vi "read_params.vi"(8 "error in (no error)":errorcluster, 11 "OPTICS in":refnum<class "OPTICS.lvclass">) -> (0 "error out":errorcluster, 2 "params":T1={"min_samples"=5.0, "max_eps"=inf, "metric"="euclidean", "p"=2.0, "cluster_method"="xi", "eps"={"eps_type"="None", "eps_float"=0.0}, "xi"=0.05, "predecessor_correction"=TRUE, "min_cluster_size"={"min_cluster_size_type"="None", "min_cluster_size_int"=1.0, "min_cluster_size_float"=0.0}, "algorithm"="auto", "leaf_size"=30.0, "n_jobs"=1.0}, 3 "OPTICS out":refnum<class "OPTICS.lvclass">)   [LabVIEW 2020, in "OPTICS.lvclass"]
uses:
  OPTICS.lvclass
  Controls/optics_params.ctl
  OPTICS.lvclass/OPTICS.ctl
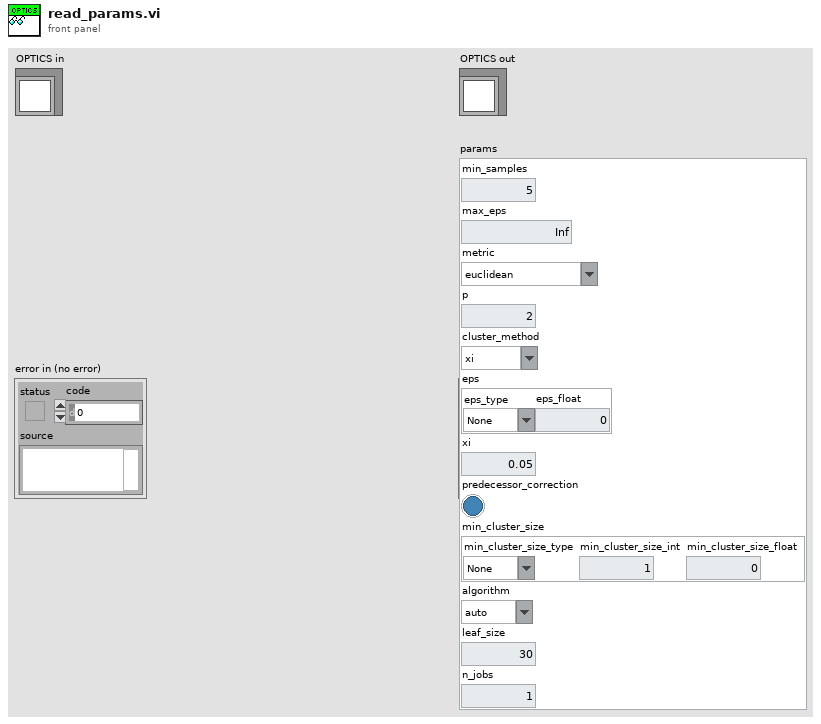
[diagram p1: front panel]
types:
  T1 = typedef "optics_params.ctl" = cluster{"min_samples":dbl, "max_eps":dbl, "metric":string, "p":dbl, "cluster_method":string, "eps":cluster{"eps_type":string, "eps_float":dbl}, "xi":dbl, "predecessor_correction":bool, "min_cluster_size":cluster{"min_cluster_size_type":string, "min_cluster_size_int":dbl, "min_cluster_size_float":dbl}, "algorithm":string, "leaf_size":dbl, "n_jobs":dbl}
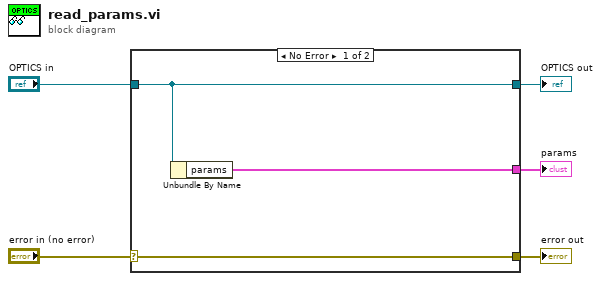
[diagram p0: block diagram]
diagram:
  n1 = case shown="No Error" "error in (no error)" {
    selector: "error in (no error)" -> [w8 w9]
    tunnel: [w8 w9] -> w4
    tunnel: [w7 w10] -> w2
    tunnel: "OPTICS in" -> [w7 w10]
    tunnel: [w6 _] -> w1
    frame No Error {
      n2 = Unbundle By Name(w7) -> ("params"=w6:T1)
    }
    frame Error {
    }
  }
  "error out" <- w4
  "OPTICS out" <- w2
  "params" <- w1
